vi "Write Single element To XL.vi"(8 "error in":errorcluster, 9 "Write/Read Cell":T1={"Cell Range"="", "Data 2D"=[], "Select Sheet"="", "1 Data"="", "Data 1D"=[], "Font col"=0, "Bold"=TRUE, "Font Size"=18, "Inside lines"=FALSE}, 10 "Work Sheet":refnum<k7>) -> (0 "error out":errorcluster, 2 "Work Sheet":refnum<k7>)   [LabVIEW 2017]
uses:
  controls/read.write.ctl
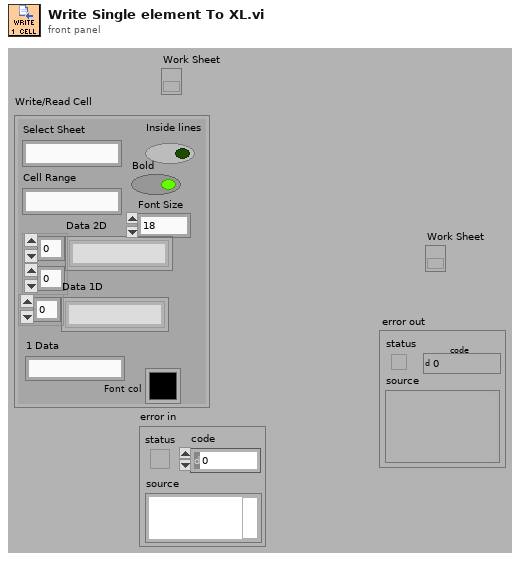
[diagram p1: front panel]
types:
  T1 = typedef "read.write.ctl" = cluster{"Cell Range":string, "Data 2D":string[][], "Select Sheet":string, "1 Data":string, "Data 1D":string[], "Font col":u32, "Bold":bool, "Font Size":i32, "Inside lines":bool}
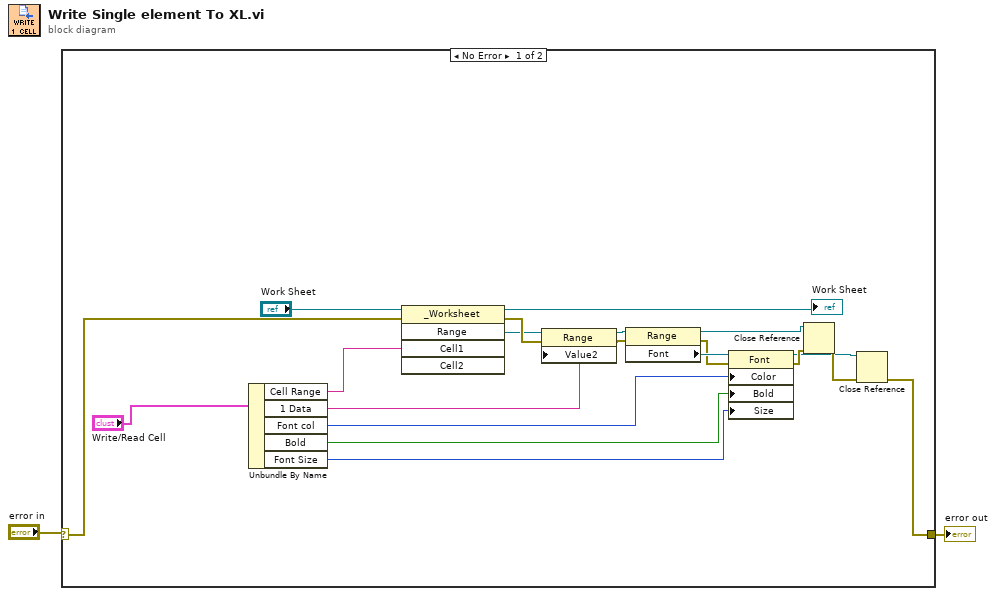
[diagram p0: block diagram]
diagram:
  n1 = case shown="No Error" "error in" {
    selector: "error in" -> [w22 w23]
    tunnel: [w8 w23] -> w1
    frame No Error {
      n2 = Unbundle By Name("Write/Read Cell") -> ("Cell Range"=w18:string, "1 Data"=w3:string, "Font col"=w7:u32, "Bold"=w5:bool, "Font Size"=w6:i32)
      n3 = invoke class="_Worksheet" method="Range"(reference="Work Sheet", error in=w22, "Cell1"=w18) -> (reference out=→"Work Sheet":refnum<k7>, error out=w21:errorcluster, "Range"=w17:refnum<k7>)  [unwired: 2 in, 2 out]
      n4 = property class="Range"(reference=w17, error in=w21, "Value2"=w3) -> (reference out=w16:refnum<k7>, error out=w14:errorcluster)
      n5 = property class="Range"(reference=w16, error in=w14) -> (reference out=w9:refnum<k7>, error out=w13:errorcluster, "Font"=w15:refnum<k7>)
      n6 = property class="Font"(reference=w15, error in=w13, "Color"=w7, "Bold"=w5, "Size"=w6) -> (reference out=w10:refnum<k7>, error out=w12:errorcluster)
      n7 = Close Reference(reference=w9, error in (no error)=w12) -> (error out=w11:errorcluster)
      n8 = Close Reference(reference=w10, error in (no error)=w11) -> (error out=w8:errorcluster)
    }
    frame Error {
    }
  }
  "error out" <- w1
